vi "ClearErrors.vi"(8 "ErrorIn Array":errorcluster[](array[cluster])) -> (0 "Error Out Array":errorcluster[](array[cluster]))   [LabVIEW 2018, in "NISTErrorLib.lvlib"]
doc: "Clears errors/warnings that occurred."
uses:
  NISTErrorLib.lvlib
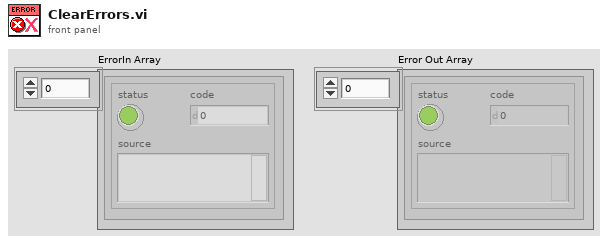
[diagram p1: front panel]
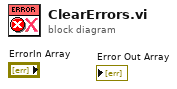
[diagram p0: block diagram]
diagram:
